vi "verify acquisition parameters.vi"(8 "error in (no error)":errorcluster, 11 "Channel in":refnum<class "Channel.lvclass">) -> (0 "error out":errorcluster, 3 "Channel out":refnum<class "Channel.lvclass">)   [LabVIEW 2018, in "Channel.lvclass"]
uses:
  Channel.lvclass
  Channel.lvclass/Channel.ctl
  Simulated_CCD_Camera/Simulated Camera.lvclass
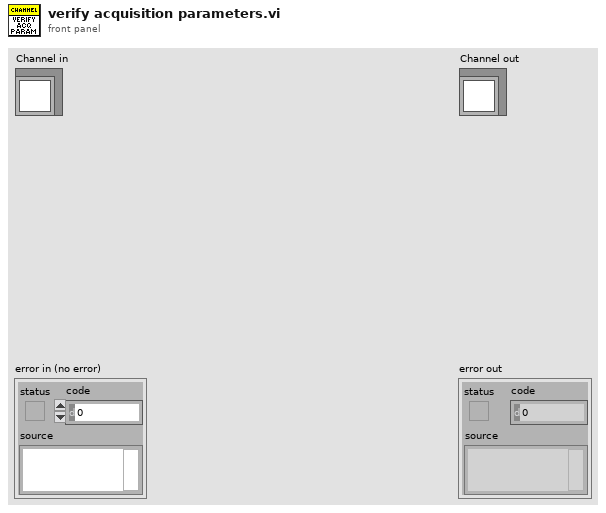
[diagram p1: front panel]
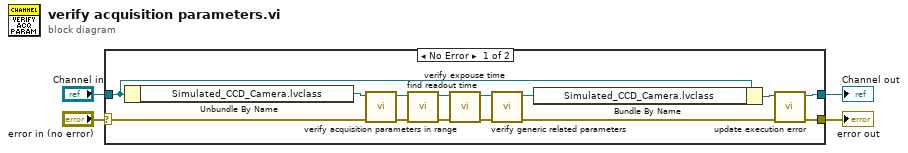
[diagram p0: block diagram]
diagram:
  n1 = case shown="No Error" "error in (no error)" {
    selector: "error in (no error)" -> [w10 w20]
    tunnel: [w6 w20] -> w3
    tunnel: [w7 w19] -> w1
    tunnel: "Channel in" -> [w11 w19]
    frame No Error {
      n2 = Unbundle By Name(w11) -> ("Simulated_CCD_Camera.lvclass"=w12:refnum<class "Simulated Camera.lvclass">)
      n3 = call "verify acquisition parameters in range.vi"("error in (no error)"=w10, "Simulated_CCD_Camera in"=w12) -> ("error out"=w13:errorcluster, "Simulated_CCD_Camera out"=w14:refnum<class "Simulated Camera.lvclass">)  [unwired: 8 in]
      n4 = call "find readout time.vi"("error in (no error)"=w13, "Simulated_CCD_Camera in"=w14) -> ("error out"=w17:errorcluster, "Simulated_CCD_Camera out"=w18:refnum<class "Simulated Camera.lvclass">)  [unwired: 8 in]
      n5 = call "verify expouse time.vi"("error in (no error)"=w17, "Simulated_CCD_Camera in"=w18) -> ("error out"=w16:errorcluster, "Simulated_CCD_Camera out"=w15:refnum<class "Simulated Camera.lvclass">)  [unwired: 8 in]
      n6 = call "verify generic related parameters.vi"("error in (no error)"=w16, "Simulated_CCD_Camera in"=w15) -> ("error out"=w5:errorcluster, "Simulated_CCD_Camera out"=w9:refnum<class "Simulated Camera.lvclass">)  [unwired: 8 in]
      n7 = Bundle By Name(cluster=w11, "Simulated_CCD_Camera.lvclass"=w9) -> (w8:refnum<class "Channel.lvclass">)
      n8 = call "update execution error.vi"("error in (no error)"=w5, "Channel in"=w8) -> ("error out"=w6:errorcluster, "Channel out"=w7:refnum<class "Channel.lvclass">)  [unwired: 8 in]
    }
    frame Error {
    }
  }
  "error out" <- w3
  "Channel out" <- w1
